vi "CMFB diagnostic (RT).vi"() -> ()   [LabVIEW 2019]
uses:
  <vilib>/FPGAPlugInAG/sbRIO-9627/niLvFpga_Open_sbRIO-9627.vi
  <vilib>/rvi/interface/common/dynamic/niFpgaDynamicAddResources.vi
  <vilib>/Utility/error.llb/Error Cluster From Error Code.vi
  <vilib>/rvi/errors/niLvFpgaAdjustHostInterfaceError.vi
  <vilib>/rvi/interface/nirviOpenFPGA/nirviOpenFPGA.xnode
  FPGA Bitfiles/tisbrio_FPGATarget2_CMFBdiagnostic_APBZv+3FN24.lvbitx
  <vilib>/rvi/interface/nirviReadWriteControl/nirviReadWriteControl.xnode
  NiFpgaLv.dll
  <vilib>/rvi/interface/Simulation/niFpgaSimulationCallBeginRW.vi
panel:
  out "flow freq":fxp<+/-,28,17>
  out "diag freq":fxp<+/-,32,32>
  out "Diagnostic (duty)":fxp<+/-,28,17>
  in  "Wait Low (ms)":u32
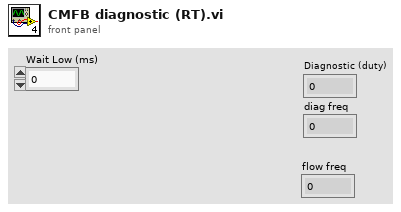
[diagram p1: front panel]
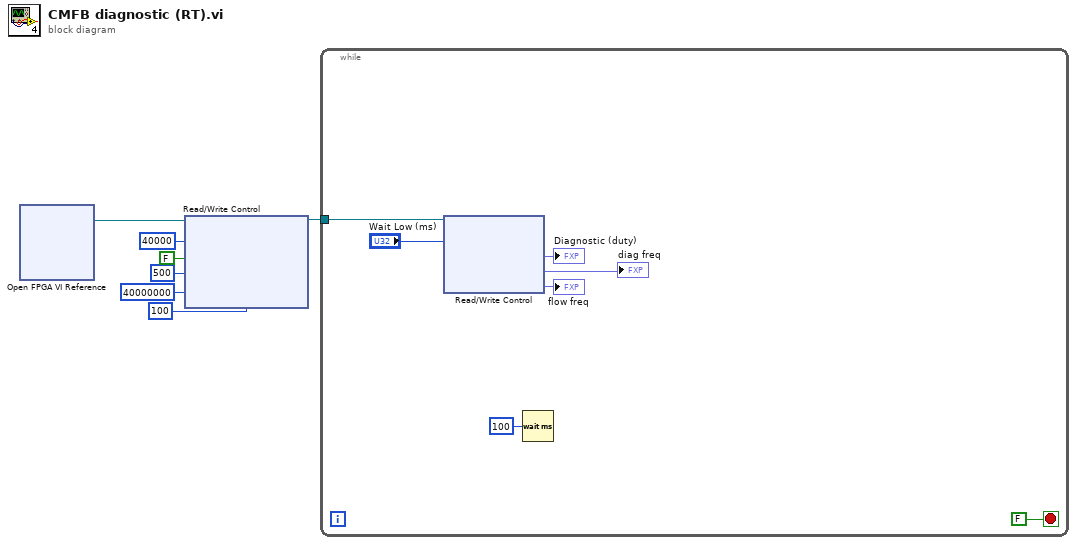
[diagram p0: block diagram]
diagram:
  n1 = xnode "Open FPGA VI Reference"() -> ("FPGA VI Reference Out"=w7:refnum<k20>)  [unwired: 2 in, 1 out]
  n2 = xnode "Read/Write Control"("FPGA VI Reference In"=w7, "Diagnostic Freq Coeff"=40000, "Invert Diagnostic"=FALSE, "Diagnostic Filter"=u16 500, "Max Period (ticks)"=u32 40000000, "Wait High (ms)"=u32 100) -> ("FPGA VI Reference Out"=w2:refnum<k20>)  [unwired: 1 in, 1 out]
  n3 = while {
    tunnel: w2 -> [w13]
    stop <- FALSE stop-if-true
    n4 = xnode "Read/Write Control"("FPGA VI Reference In"=w13, "Wait Low (ms)"="Wait Low (ms)") -> ("Diagnostic (duty)"=→"Diagnostic (duty)":fxp<+/-,28,17>, "diag freq"=→"diag freq":fxp<+/-,32,32>, "flow freq"=→"flow freq":fxp<+/-,28,17>)  [unwired: 1 in, 2 out]
    n5 = Wait (ms)(milliseconds to wait=u32 100) -> ()  [unwired: 1 out]
  }
